vi "数值比较选择函数.vi"() -> ()   [LabVIEW 2022 SP3]
doc: "本VI是为《我和LabVIEW》一书编写的示例。\n关于本书的介绍请参考网页：\nhttp://ruanqizhen.spaces.live.com/blog/cns!5852D4F797C53FB6!4310.entry"
panel:
  in  "b":i32
  in  "a":i32
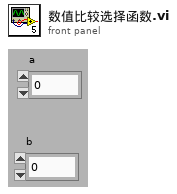
[diagram p1: front panel]
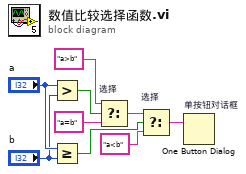
[diagram p0: block diagram]
diagram:
  n1 = Greater?(x="a", y="b") -> (0:w7:bool)
  n2 = Greater Or Equal?(x="a", y="b") -> (x >= y?=w4:bool)
  n3 = Select "选择"(t="a>b", s=w7, f="a=b") -> (s? t:f=w3:string)
  n4 = Select "选择"(t=w3, s=w4, f="a<b") -> (s? t:f=w1:string)
  n5 = One Button Dialog "单按钮对话框"(message=w1) -> ()  [unwired: 2 out]
